vi "SUB_ASCII_2_Char.vi"(3 "Input String":string="0ABCDEF") -> (1 "Char":string)   [LabVIEW 2011]
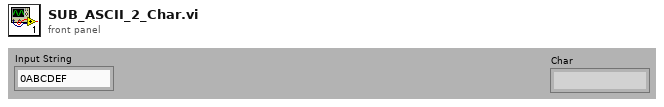
[diagram p1: front panel]
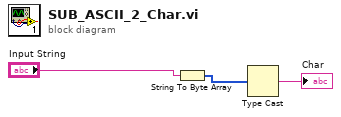
[diagram p0: block diagram]
diagram:
  n1 = String To Byte Array(string="Input String") -> (unsigned byte array=w2:u8[])
  n2 = Type Cast(x=w2) -> (*(type *) &x=→"Char":string)  [unwired: 1 in]
